vi "PathPlanner_RotationTarget_Equals.vi"(9 "Other GoalEndState":T1={"target"={"VALUE"=0.0, "COS"=1.0, "SIN"=0.0}, "WaypointRelativePosition"=0.0, "Exists"=FALSE} {"target"."SIN" format="%13.4f"; "target"."COS" format="%13.4f"; "target"."VALUE" format="%13.4f"}, 11 "RotationTarget":T1={"target"={"VALUE"=0.0, "COS"=1.0, "SIN"=0.0}, "WaypointRelativePosition"=0.0, "Exists"=FALSE} {"target"."SIN" format="%13.4f"; "target"."COS" format="%13.4f"; "target"."VALUE" format="%13.4f"}) -> (3 "Equal":bool)   [LabVIEW 2019, in "PathPlanner24.lvlib"]
doc: "Determine if two rotation targets are equal\n\nInputs: \n - RotationTarget - cluster - defined rotation target data structure\n - OtherRotationTarget - cluster - defined rotation target data structure\n\nOutputs:\n - Equal - boolean - TRUE if both rotation targets are the same"
uses:
  PathPlanner24.lvlib
  TypeDef/PathPlannerRotationTarget.ctl
  <vilib>/Rock Robotics/WPI/ThirdParty/JAS_Junk/TrajLib/TypeDef/ROTATION2D.ctl
  <vilib>/Rock Robotics/WPI/ThirdParty/JAS_Junk/TrajLib/Util_CalcDist.vi
  <vilib>/Rock Robotics/WPI/ThirdParty/JAS_Junk/TrajLib/Trajectory_Library.lvlib
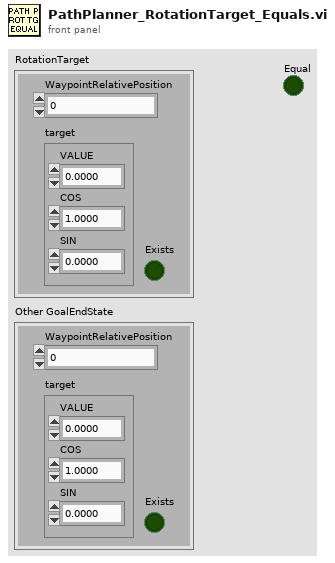
[diagram p1: front panel]
types:
  T1 = typedef "PathPlanner24.lvlib/PathPlannerRotationTarget.ctl" = cluster{"target":T2, "WaypointRelativePosition":dbl, "Exists":bool}
  T2 = typedef "Trajectory_Library.lvlib/ROTATION2D.ctl" = cluster{"VALUE":dbl, "COS":dbl, "SIN":dbl}
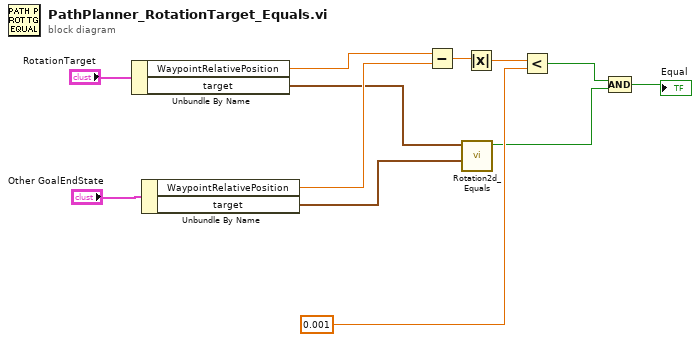
[diagram p0: block diagram]
diagram:
  n1 = Unbundle By Name("RotationTarget") -> ("WaypointRelativePosition"=w10:dbl, "target"=w3:T2)
  n2 = Unbundle By Name("Other GoalEndState") -> ("WaypointRelativePosition"=w9:dbl, "target"=w2:T2)
  n3 = Subtract(x=w10, y=w9) -> (x-y=w8:dbl)
  n4 = call <vilib>:"Rotation2d_Equals.vi"("other ROTATION"=w2, "in ROTATION"=w3) -> ("Equals"=w1:bool)  [unwired: 9 in]
  n5 = Absolute Value(x=w8) -> (abs(x)=w7:dbl)
  n6 = Less?(x=w7, y=0.001) -> (x < y?=w6:bool)
  n7 = Compound Arithmetic op=AND(w6, w1) -> (→"Equal":bool)
